vi "FTW-Subscriber-Destroy.vi"(0 "FTW-Subscription In":refnum<class "FTW-Subscriber.lvclass">, 11 "error in":errorcluster) -> (15 "error out":errorcluster)   [LabVIEW 2013, in "FTW-Subscriber.lvclass"]
uses:
  FTW-Subscriber.lvclass
  FTW-Subscriber.lvclass/FTW-Subscriber.ctl
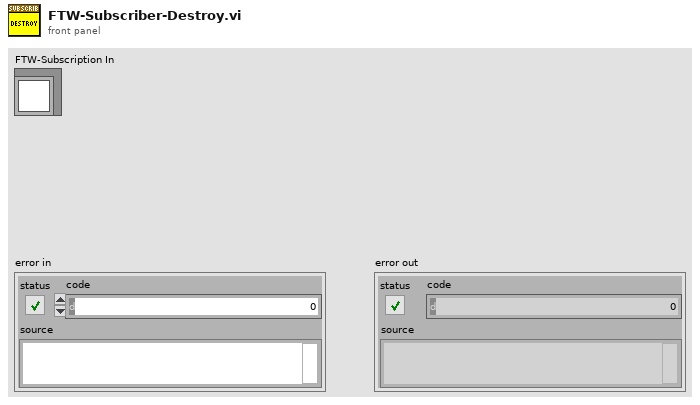
[diagram p1: front panel]
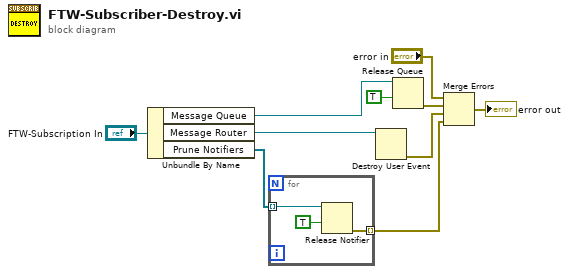
[diagram p0: block diagram]
diagram:
  n1 = Unbundle By Name("FTW-Subscription In") -> ("Message Queue"=w3:refnum<queue>, "Message Router"=w7:refnum<user-event>, "Prune Notifiers"=w5:refnum<notifier>[])
  n2 = for {
    tunnel: w5 -> [w13] mode=indexing
    tunnel: [w11] -> w4 mode=indexing
    n3 = Release Notifier(notifier=w13, force destroy? (F)=TRUE) -> (error out=w11:errorcluster)  [unwired: 1 in, 2 out]
  }
  n4 = Destroy User Event(user event=w7) -> (error out=w6:errorcluster)  [unwired: 1 in]
  n5 = Release Queue(queue=w3, force destroy? (F)=TRUE) -> (error out=w1:errorcluster)  [unwired: 1 in, 2 out]
  n6 = Merge Errors("error in", w1, w6, w4) -> (→"error out":errorcluster)
